vi "power conversion.vi"(8 "error in (no error)":errorcluster, 11 "AOTF in":refnum<class "AOTF.lvclass">) -> (0 "error out":errorcluster, 2 "Power voltage out":dbl, 3 "AOTF out":refnum<class "AOTF.lvclass">)   [LabVIEW 2012, in "AOTF.lvclass"]
uses:
  AOTF.lvclass
  Controls/laser line ring.ctl
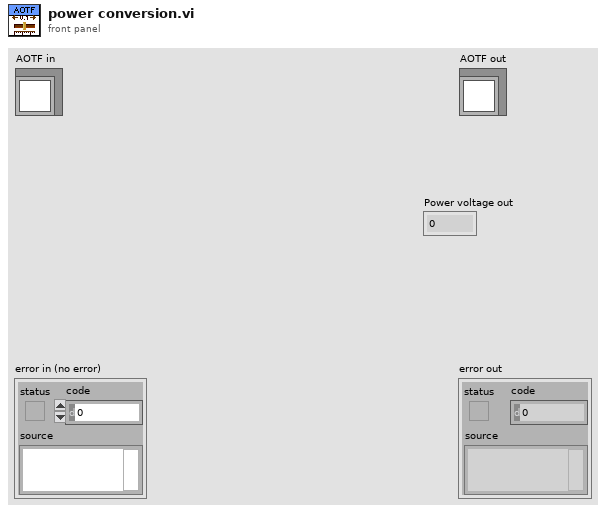
[diagram p1: front panel]
types:
  T1 = typedef "AOTF.lvclass/laser line ring.ctl" = u8
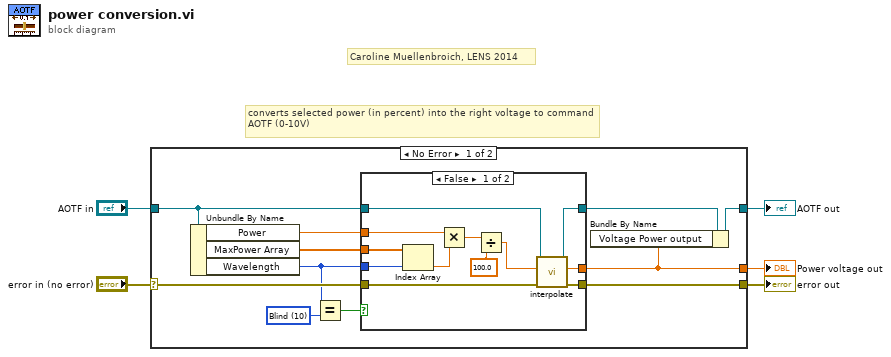
[diagram p0: block diagram]
diagram:
  # "converts selected power (in percent) into the right voltage to command AOTF (0-10V)"
  # "Caroline Muellenbroich, LENS 2014"
  n1 = case shown="No Error" "error in (no error)" {
    selector: "error in (no error)" -> [w16 w32]
    tunnel: [w15 w32] -> w4
    tunnel: [w10 w31] -> w2
    tunnel: "AOTF in" -> [w12 w31]
    tunnel: [w9 _] -> w1
    frame No Error {
      w7 = T1 10 items=["Blind"=10, "405nm"=0, "445nm"=5, "491nm"=1, "515nm"=2, "561nm"=3] ("y")
      n2 = Unbundle By Name(w12) -> ("Power"=w14:dbl, "MaxPower Array"=w13:dbl[], "Wavelength"=w8:T1)
      n3 = Equal?(x=w8, y=w7) -> (x = y?=w6:bool)
      n4 = case shown="False" w6 {
        tunnel: w16 -> [w28 w29]
        tunnel: [w27 w29] -> w15
        tunnel: w14 -> [w26 _]
        tunnel: w13 -> [w23 _]
        tunnel: w12 -> [w21 w30]
        tunnel: [w19 w30] -> w11
        tunnel: [w18 _] -> w9
        tunnel: w8 -> [w17 _]
        frame False {
          n5 = Index Array(array=w23, index=w17) -> (element=w22:dbl)
          n6 = Multiply(x=w26, y=w22) -> (x*y=w25:dbl)
          n7 = Divide(x=w25, y=100.0) -> (x/y=w20:dbl)
          n8 = call-dynamic "interpolate.vi"("error in (no error)"=w28, "Power in"=w20, "AOTF in"=w21) -> ("error out"=w27:errorcluster, "Power voltage out"=w18:dbl, "AOTF out"=w19:refnum<class "AOTF.lvclass">)  [unwired: 6 in]
        }
        frame True {
        }
      }
      n9 = Bundle By Name(cluster=w11, "Voltage Power output"=w9) -> (w10:refnum<class "AOTF.lvclass">)
    }
    frame Error {
    }
  }
  "error out" <- w4
  "AOTF out" <- w2
  "Power voltage out" <- w1
